vi "Handle Last Ack Core.vi"(4 "error in":errorcluster, 6 "Last Ack":refnum<class "Last Ack.lvclass">, 7 "Controller in":refnum<class "Controller.lvclass">) -> (0 "error out":errorcluster, 3 "Controller out":refnum<class "Controller.lvclass">)   [LabVIEW 2014, in "Controller.lvlib" / "Controller.lvclass"]
doc: "This override of the Handle Last Ack Core keeps the controller alive until all nested actors have reported back as closed. Once no remaining nested actor enqueuers are alive, the controller will send a stop message to itself."
uses:
  Controller.lvclass
  <vilib>/ActorFramework/LastAck/Last Ack.lvclass
  Controller.lvclass/Controller.ctl
  <vilib>/ActorFramework/Actor/Actor.lvclass/Actor.ctl
  <vilib>/ActorFramework/Message Enqueuer/Message Enqueuer.lvclass/Message Enqueuer.ctl
  <vilib>/ActorFramework/Message Enqueuer/Init from Existing Queue.vi
  <vilib>/ActorFramework/Message Enqueuer/Enqueue.vi
  <vilib>/ActorFramework/Message Priority Queue/Priority Enqueue.vi
  <vilib>/ActorFramework/Stop Msg/Stop Msg.lvclass
  <vilib>/ActorFramework/Message Enqueuer/Message Enqueuer.lvclass
  <vilib>/ActorFramework/Actor/Actor.lvclass
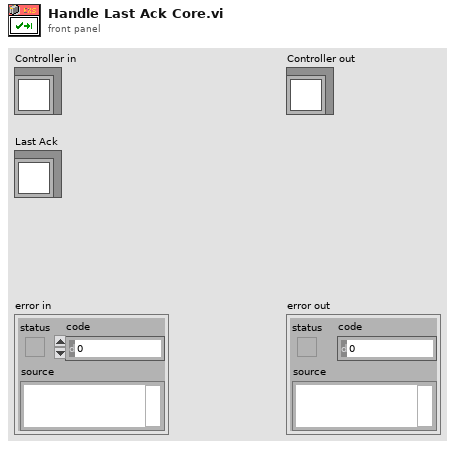
[diagram p1: front panel]
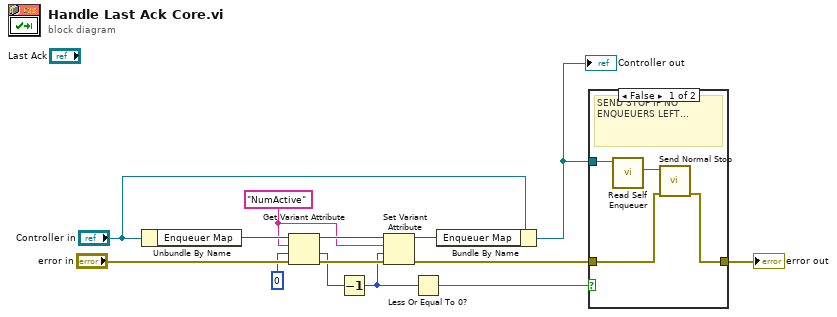
[diagram p0: block diagram]
diagram:
  w3 = "NumActive" ("name")
  n1 = Unbundle By Name("Controller in") -> ("Enqueuer Map"=w14:variant)
  n2 = Get Variant Attribute(Variant=w14, name=w3, default value (empty Variant)=i16 0, error in="error in") -> (duplicate Variant=w13:variant, value=w1:i16, error out=w12:errorcluster)  [unwired: 1 out]
  n3 = Decrement(x=w1) -> (x-1=w7:i16)
  n4 = Set Variant Attribute(Variant=w13, name=w3, value=w7, error in=w12) -> (Variant out=w9:variant, error out=w5:errorcluster)  [unwired: 1 out]
  n5 = Less Or Equal To 0?(x=w7) -> (x <= 0?=w6:bool)
  n6 = Bundle By Name(cluster="Controller in", "Enqueuer Map"=w9) -> (w8:refnum<class "Controller.lvclass">)
  "Controller out" <- w8
  n7 = case shown="False" w6 {
    tunnel: w8 -> [w17 _]
    tunnel: w5 -> [w16 w19]
    tunnel: [w15 w19] -> w4
    frame False {
      # "SEND STOP IF NO ENQUEUERS LEFT..."
      n8 = call <vilib>:"Read Self Enqueuer.vi"("Actor"=w17) -> ("Self Enqueuer"=w18:refnum<class "Message Enqueuer.lvclass">)  [unwired: 10 in]
      n9 = call <vilib>:"Send Normal Stop.vi"("error in (no error)"=w16, "Message Enqueuer"=w18) -> ("error out"=w15:errorcluster)  [unwired: 9 in]
    }
    frame True {
    }
  }
  "error out" <- w4
